vi "SL2_AD_DLL_List_Devices.vi"(4 "error in":errorcluster, 6 "dev_type":T1, 7 "dll path in":path) -> (0 "error out":errorcluster, 1 "devices":string[](array[string]), 3 "dll path out":path)   [LabVIEW 2020]
uses:
  DEFINITIONS/DEF_dev_type.ctl
  DEFINITIONS/DEF_T_error_enum.ctl
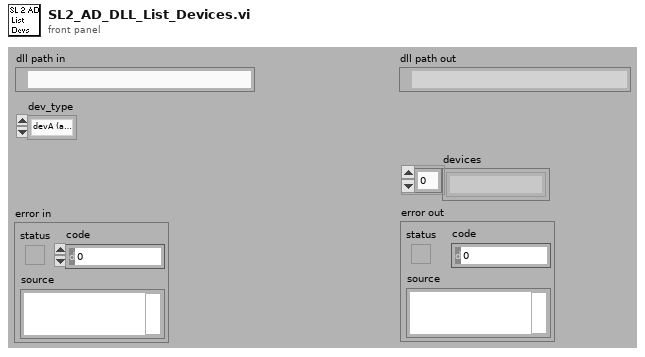
[diagram p1: front panel]
types:
  T1 = typedef "DEF_dev_type.ctl" = enum32{"devA (analyzer)", "devD (detector)"}
  T2 = typedef "DEF_T_error_enum.ctl" = u32
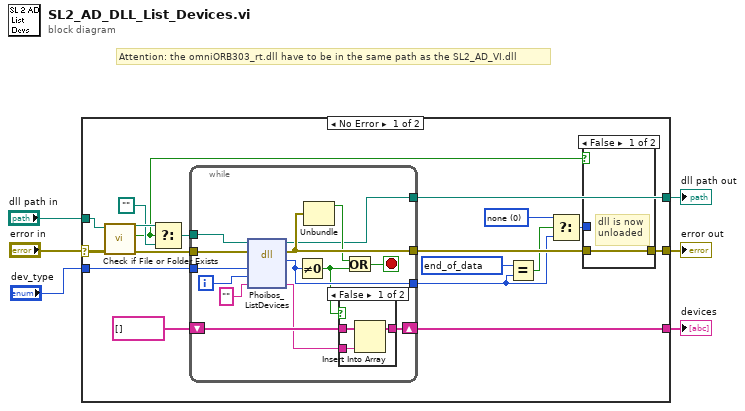
[diagram p0: block diagram]
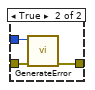
[diagram p2: hidden frame]
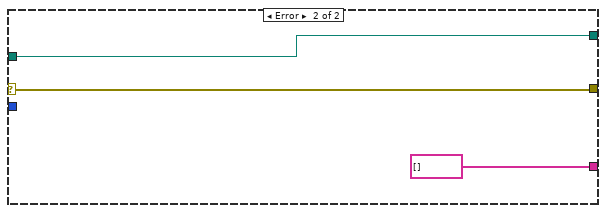
[diagram p4: hidden frame]
diagram:
  # "Attention: the omniORB303_rt.dll have to be in the same path as the SL2_AD_VI.dll"
  n1 = case shown="No Error" "error in" {
    selector: "error in" -> [w22 w48]
    tunnel: [w24 string[] [] ("Array")] -> w6
    tunnel: [w18 w48] -> w1
    tunnel: [w23 w49] -> w5
    tunnel: "dll path in" -> [w21 w49]
    tunnel: "dev_type" -> [w20 _]
    frame No Error {
      w14 = T2 8388608 items=["none"=0, "busy"=65536, "error"=131072, "parameter"=262144, "locked"=524288, "sync"=1048576, "connection"=2097152, "internal"=4194304, "end_of_data"=8388608] ("DEF_T_error_enum")
      w16 = T2 0 items=["none"=0, "busy"=65536, "error"=131072, "parameter"=262144, "locked"=524288, "sync"=1048576, "connection"=2097152, "internal"=4194304, "end_of_data"=8388608] ("DEF_T_error_enum")
      n2 = call <vilib>:"Check if File or Folder Exists.vi"("error in (no error)"=w22, "path"=w21) -> ("error out"=w12:errorcluster, "file or folder exists?"=w7:bool, "dup path"=w10:path)  [unwired: 7 in]
      n3 = Select(t=w10, s=w7, f=path "") -> (s? t:f=w9:path)
      n4 = while {
        tunnel: [w40] -> w13
        tunnel: [w33] -> w19
        shift-right: [w39] -> w24
        shift-left: string[] [] ("Array") -> [w38]
        tunnel: w9 -> [w36]
        tunnel: w12 -> [w31]
        tunnel: [w30] -> w23
        tunnel: w20 -> [w29]
        i -> [w41]
        stop <- w35 stop-if-true
        n5 = dll-call lib="C:/Programme/SPECS/SpecsLab2/programming/LabView7.1/SL2_AD_VI.dll" fn="Phoibos_ListDevices"(path in=w36, error in=w31, "dev_type"=w29, "index"=w41, "deviceID"="") -> (path out=w30:path, error out=w33:errorcluster, "error_code"=w40:u32, "deviceID"=w37:string)  [unwired: 3 in]
        n6 = Not Equal To 0?(x=w40) -> (x != 0?=w34:bool)
        n7 = Unbundle(w33) -> ("status"=w32:bool)  [unwired: 2 out]
        n8 = case shown="False" w34 {
          tunnel: [w45 w46] -> w39
          tunnel: w38 -> [w44 w46]
          tunnel: w37 -> [w43 _]
          frame False {
            n9 = Insert Into Array(array=w44, new element=w43) -> (w45:string[])  [unwired: 1 in]
          }
          frame True {
          }
        }
        n10 = Or(x=w32, y=w34) -> (x .or. y?=w35:bool)
      }
      n11 = Equal?(x=w14, y=w13) -> (x = y?=w15:bool)
      n12 = Select(t=w16, s=w15, f=w13) -> (s? t:f=w17:T2)
      n13 = case shown="False" w7 {
        tunnel: w19 -> [w25 w28]
        tunnel: [w25 w27] -> w18
        tunnel: w17 -> [_ w26]
        frame False {
          # "dll is now\nunloaded"
        }
        frame True {
          n14 = call "GenerateError.vi"("error in"=w28, "error_code"=w26) -> ("error out"=w27:errorcluster)  [unwired: 9 in]
        }
      }
    }
    frame Error {
    }
  }
  "devices" <- w6
  "error out" <- w1
  "dll path out" <- w5
